vi "Configure Buffer Size (U64).vi"(7 "FIFO Type":T1, 8 "error in":errorcluster, 10 "Buffer Size":u32=1000000 format="%.0p", 11 "FPGA VI Reference In":refnum<k20>) -> (0 "error out":errorcluster, 3 "FPGA VI Reference Out":refnum<k20>)   [LabVIEW 2012]
doc: "This start acquisition by switching OFF and ON \"Arm Acquire button\".\nThis VI also starts DMA FIFO."
uses:
  <userlib>/FlexRIO Host Library/FlexRIO Host API/Acquire/FIFO Type.ctl
  <vilib>/Utility/error.llb/Error Cluster From Error Code.vi
  <vilib>/rvi/interface/nirviMethod/nirviMethod.xnode
  <vilib>/rvi/errors/niLvFpgaMergeErrorWithErrorCode.vi
  <vilib>/FPGAPlugInAG/Dynamic/niLvFpga_ConfigureFifo_Dynamic.vi
  <vilib>/FPGAPlugInAG/Dynamic/niLvFpga_StartFifo_Dynamic.vi
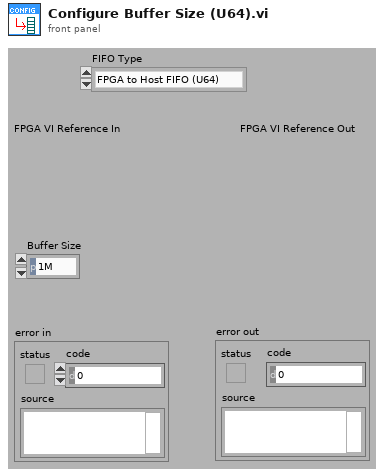
[diagram p1: front panel]
types:
  T1 = typedef "FIFO Type.ctl" = enum16{"FPGA to Host FIFO (U64)", "Generic", "FPGA to Host FIFO (U32)"}
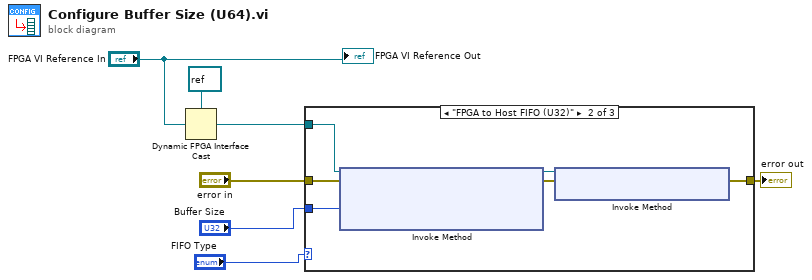
[diagram p0: block diagram]
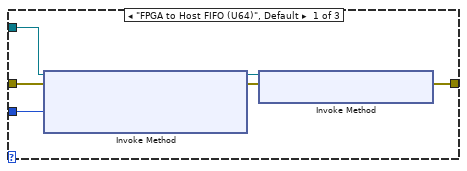
[diagram p2: hidden frame]
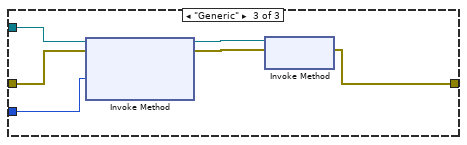
[diagram p3: hidden frame]
diagram:
  n1 = Dynamic FPGA Interface Cast(Session In=refnum<k20> refnum ("Type"), Type="FPGA VI Reference In") -> (Session Out=w3:refnum<k20>)
  n2 = case shown="\"FPGA to Host FIFO (U32)\"" "FIFO Type" {
    tunnel: "Buffer Size" -> [w13 w19 w21]
    tunnel: "error in" -> [w12 w18 w22]
    tunnel: [w11 w17 w20] -> w5
    tunnel: w3 -> [w10 w16 w23]
    frame "FPGA to Host FIFO (U64)", Default {
      n3 = xnode "Invoke Method"("FPGA VI Reference In"=w10, "error in"=w12, "Requested Depth"=w13) -> ("FPGA VI Reference Out"=w9:refnum<k20>, "error out"=w8:errorcluster)  [unwired: 1 out]
      n4 = xnode "Invoke Method"("FPGA VI Reference In"=w9, "error in"=w8) -> ("error out"=w11:errorcluster)  [unwired: 1 out]
    }
    frame "FPGA to Host FIFO (U32)" {
      n5 = xnode "Invoke Method"("FPGA VI Reference In"=w16, "error in"=w18, "Requested Depth"=w19) -> ("FPGA VI Reference Out"=w15:refnum<k20>, "error out"=w14:errorcluster)  [unwired: 1 out]
      n6 = xnode "Invoke Method"("FPGA VI Reference In"=w15, "error in"=w14) -> ("error out"=w17:errorcluster)  [unwired: 1 out]
    }
    frame "Generic" {
      n7 = xnode "Invoke Method"("FPGA VI Reference In"=w23, "error in"=w22, "Requested Depth"=w21) -> ("FPGA VI Reference Out"=w25:refnum<k20>, "error out"=w24:errorcluster)  [unwired: 1 out]
      n8 = xnode "Invoke Method"("FPGA VI Reference In"=w25, "error in"=w24) -> ("error out"=w20:errorcluster)  [unwired: 1 out]
    }
  }
  "error out" <- w5
  "FPGA VI Reference Out" <- "FPGA VI Reference In"
